vi "Dinero Update.vi"(8 "error in (no error)":errorcluster, 10 "Dinero":dbl, 11 "UI in":refnum<class "UI.lvclass">) -> (0 "error out":errorcluster, 3 "UI out":refnum<class "UI.lvclass">)   [LabVIEW 2021, in "UI.lvlib" / "UI.lvclass"]
uses:
  UI.lvclass
  UI.lvclass/UI.ctl
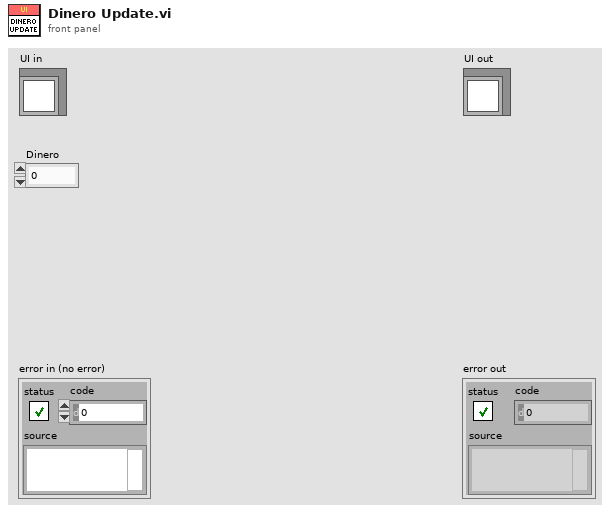
[diagram p1: front panel]
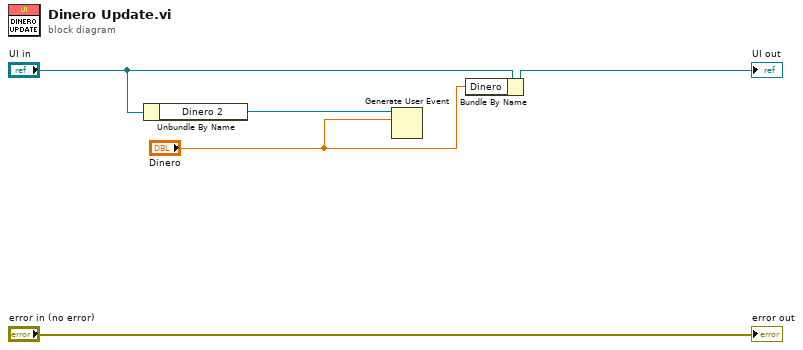
[diagram p0: block diagram]
diagram:
  n1 = Unbundle By Name("UI in") -> ("Dinero 2"=w4:refnum<user-event>)
  n2 = Generate User Event(user event=w4, event data cluster="Dinero") -> ()  [unwired: 2 in, 2 out]
  n3 = Bundle By Name(cluster="UI in", "Dinero"="Dinero") -> (→"UI out":refnum<class "UI.lvclass">)
  "error out" <- "error in (no error)"
